vi "loggingModuleStart.vi"(8 "error in (no error)":errorcluster) -> (0 "error out":errorcluster, 3 "message out":T1)   [LabVIEW 2017, in "loggingModule.lvlib"]
uses:
  loggingModule.lvlib
  programControl/Notifier/TypeDefs/notificationMessage.ctl
  programControl/Notifier/TypeDefs/notifierFGVStates.ctl
  programControl/programControl.lvlib
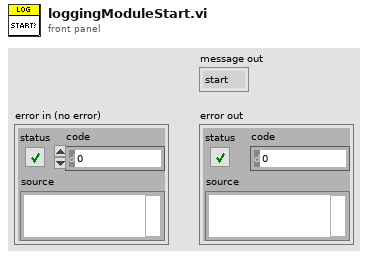
[diagram p1: front panel]
types:
  T1 = typedef "programControl.lvlib/notificationMessage.ctl" = enum16{"start", "wait", "run", "end"}
  T2 = typedef "programControl.lvlib/notifierFGVStates.ctl" = enum16{"obtain", "send", "wait for notification", "release"}
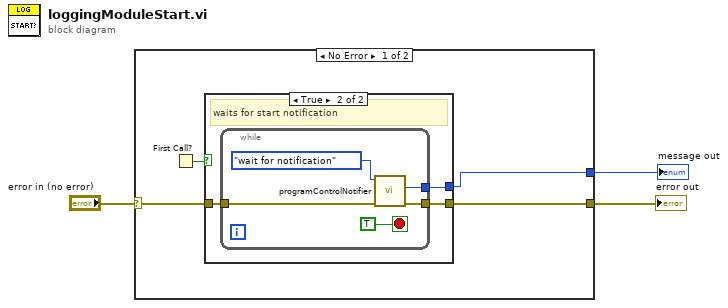
[diagram p0: block diagram]
diagram:
  n1 = case shown="No Error" "error in (no error)" {
    selector: "error in (no error)" -> [w5 w17]
    tunnel: [w7 w17] -> w3
    tunnel: [w4 _] -> w1
    frame No Error {
      n2 = First Call?() -> (First Call?: T/F=w6:bool)
      n3 = case shown="True" w6 {
        tunnel: [w8 w11] -> w7
        tunnel: [_ w10] -> w4
        tunnel: w5 -> [w8 w9]
        frame False {
        }
        frame True {
          # "waits for start notification"
          n4 = while {
            tunnel: [w14] -> w11
            tunnel: [w13] -> w10
            tunnel: w9 -> [w12]
            stop <- TRUE stop-if-true
            n5 = call "programControlNotifier.vi"("error in (no error)"=w12, "Enum"=notifierFGVStates."wait for notification") -> ("error out"=w14:errorcluster, "message out"=w13:T1)  [unwired: 8 in]
          }
        }
      }
    }
    frame Error {
    }
  }
  "error out" <- w3
  "message out" <- w1
